vi "多参数数据插入.vi"(8 "error in (no error)":errorcluster caption="错误输入（无错误）", 9 "编号":string, 10 "columns enable":T1, 11 "data in":T2) -> (0 "error out":errorcluster)   [LabVIEW 2016, in "斯坦道多参数.lvlib"]
uses:
  <vilib>/Utility/sysdir.llb/System Directory Type.ctl
  <vilib>/addons/database/Auxilliary.llb/DB Tools Parameter Info.ctl
  <vilib>/addons/database/Auxilliary.llb/DB Tools DataTypes.ctl
  <vilib>/addons/database/Auxilliary.llb/DB Tools Parameter Dir.ctl
  <vilib>/addons/database/Auxilliary.llb/DB Tools Column Info.ctl
  <vilib>/addons/database/Auxilliary.llb/DB Tools Format Datetime String (Time Stamp).vi
  <vilib>/addons/database/Connection.llb/DB Tools Open Connec (String).vi
  <vilib>/addons/database/Connection.llb/Conn Execute.vi
  <vilib>/addons/database/Recordset.llb/Rec Destroy - Connection.vi
  <vilib>/addons/database/Command.llb/Cmd Set Parameter Value (C).vi
  <vilib>/addons/database/Command.llb/Cmd Execute.vi
  <vilib>/addons/database/Recordset.llb/Rec Destroy - Command.vi
  <vilib>/addons/database/Command.llb/Cmd Delete.vi
  <vilib>/addons/database/NI_Database_API.lvlib
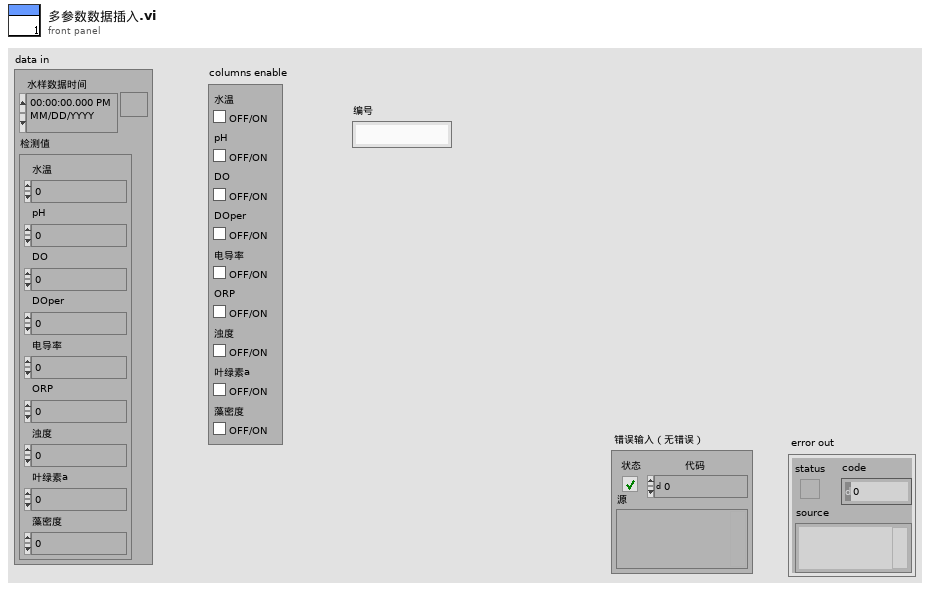
[diagram p1: front panel]
types:
  T1 = cluster{"水温":bool, "pH":bool, "DO":bool, "DOper":bool, "电导率":bool, "ORP":bool, "浊度":bool, "叶绿素a":bool, "藻密度":bool}
  T2 = cluster{"水样数据时间":timestamp, "检测值":cluster{"水温":dbl, "pH":dbl, "DO":dbl, "DOper":dbl, "电导率":dbl, "ORP":dbl, "浊度":dbl, "叶绿素a":dbl, "藻密度":dbl}}
  T3 = typedef "System Directory Type.ctl" = i32
  T4 = cluster{"水温":dbl, "pH":dbl, "DO":dbl, "DOper":dbl, "电导率":dbl, "ORP":dbl, "浊度":dbl, "叶绿素a":dbl, "藻密度":dbl}
  T5 = typedef "NI_Database_API.lvlib/DB Tools Column Info.ctl" = cluster{"column name":string, "data type":T6, "size":i32, "allow null?":bool}
  T6 = typedef "NI_Database_API.lvlib/DB Tools DataTypes.ctl" = enum16{"String", "Long (I32)", "Single (SGL)", "Double (DBL)", "Date/Time", "Binary"}
  T7 = typedef "NI_Database_API.lvlib/DB Tools Parameter Info.ctl" = cluster{"parameter name":string, "type":T6, "direction":T8, "value":variant}
  T8 = typedef "NI_Database_API.lvlib/DB Tools Parameter Dir.ctl" = enum32{"Input", "Output", "Input/Output", "Return Value"}
  T9 = typedef "NI_Database_API.lvlib/Conn ObjectReference.ctl" = refnum<k1>
  T10 = typedef "NI_Database_API.lvlib/Rec ObjectReference.ctl" = refnum<k1>
  T11 = typedef "NI_Database_API.lvlib/Cmd ObjectReference.ctl" = refnum<k1>
  T12 = typedef "NI_Database_API.lvlib/Cmd-Rec Object Reference.ctl" = refnum<k1>
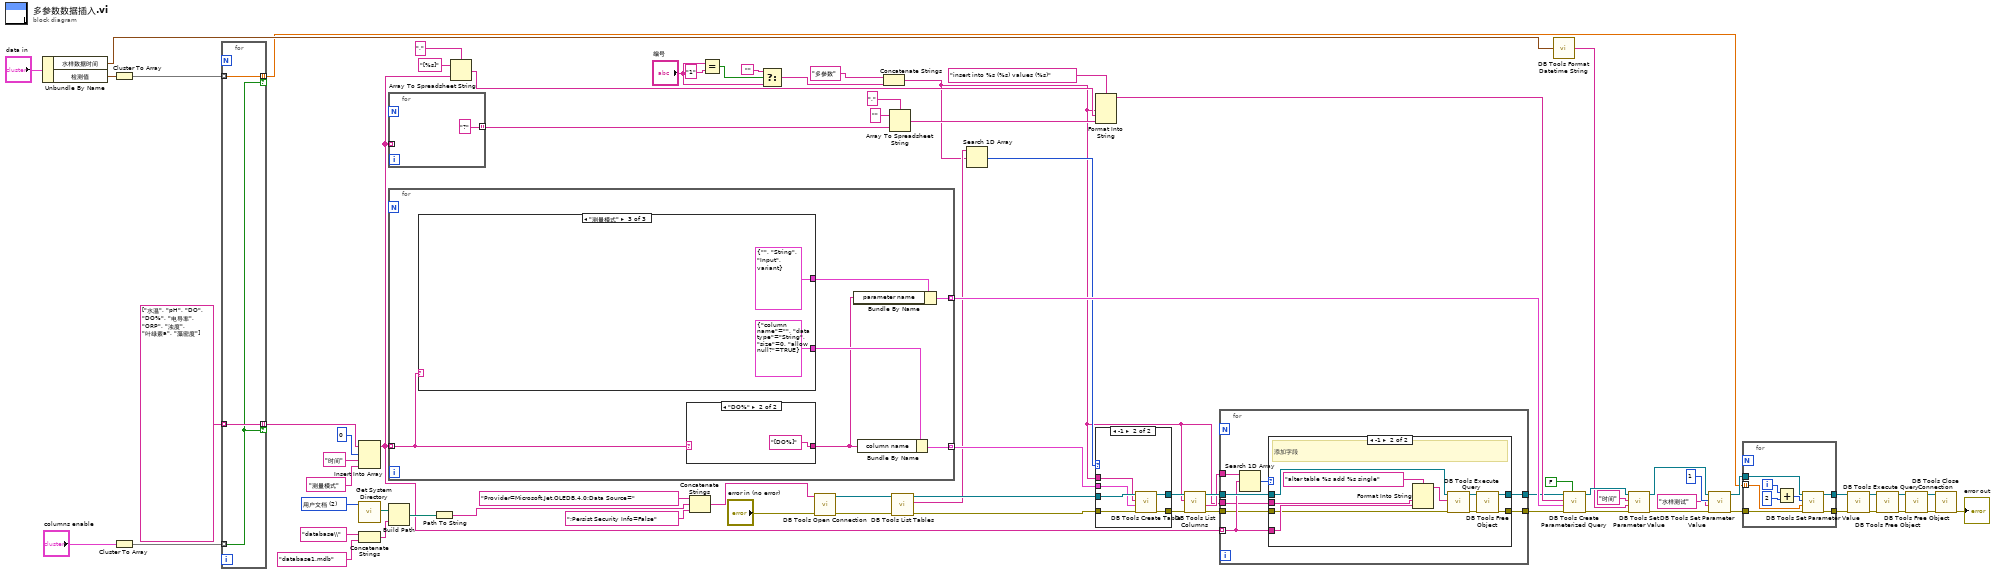
[diagram p0: block diagram]
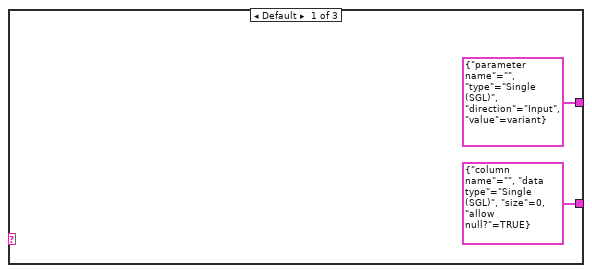
[diagram p5: hidden frame]
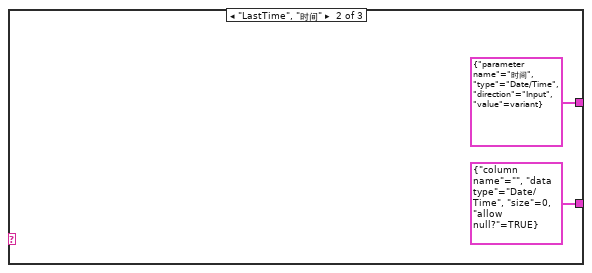
[diagram p6: hidden frame]
diagram:
  w75 = T3 2 items=["用户目录"=0, "用户桌面"=1, "用户文档"=2, "用户应用程序数据"=3, "用户设置"=4, "用户临时目录"=5, "公共文档"=6, "公共应用程序数据"=7, "公共设置"=8, "公共缓存"=13, "系统核心库"=9, "系统安装库"=10, "应用程序文件"=11, "启动盘根目录"=12] ("system directory type")
  n1 = Unbundle By Name("data in") -> ("水样数据时间"=w31:timestamp, "检测值"=w21:T4)
  n2 = Cluster To Array(cluster=w21) -> (array=w20:dbl[])
  n3 = Cluster To Array(cluster="columns enable") -> (array=w59:bool[])
  n4 = for {
    tunnel: string[] ["水温", "pH", "DO", "DO%", "电导率", "ORP", "浊度", "叶绿素a", "藻密度"] ("columns name") -> [w78] mode=indexing
    tunnel: w59 -> [w76] mode=indexing
    tunnel: [w78] -> w8 mode=indexing if=w76
    tunnel: w20 -> [w77] mode=indexing
    tunnel: [w77] -> w19 mode=indexing if=w76
  }
  n5 = Insert Into Array(array=w8, index=0 ("索引"), new element #1="时间" ("新元素/子数组"), new element #2="测量模式" ("新元素/子数组")) -> (w16:string[])
  n6 = call <vilib>:"Get System Directory.vi"("system directory type"=w75) -> ("system directory"=w73:path)  [unwired: 10 in]
  n7 = Concatenate Strings("database\\" ("condition"), "database1.mdb" ("字符串")) -> (w67:string)
  n8 = for {
    tunnel: w16 -> [_] mode=indexing
    tunnel: ["?"] -> w46 mode=indexing
  }
  n9 = for {
    tunnel: w16 -> [w81] mode=indexing
    tunnel: [w82] -> w44 mode=indexing
    tunnel: [w84] -> w43 mode=indexing
    n10 = case shown="\"测量模式\"" w81 {
      tunnel: [T7 {"parameter name"="", "type"=enum."Single (SGL)", "direction"=enum."Input", "value"=variant} ("parameter information") T7 {"parameter name"="时间", "type"=enum."Date/Time", "direction"=enum."Input", "value"=variant} ("parameter information") T7 {"parameter name"="", "type"=enum."String", "direction"=enum."Input", "value"=variant} ("parameter information")] -> w83
      tunnel: [T5 {"column name"="", "data type"=enum."Single (SGL)", "size"=0, "allow null?"=TRUE} ("column information") T5 {"column name"="", "data type"=enum."Date/Time", "size"=0, "allow null?"=TRUE} ("column information") T5 {"column name"="", "data type"=enum."String", "size"=0, "allow null?"=TRUE} ("column information")] -> w85
      frame Default {
      }
      frame "LastTime", "时间" {
      }
      frame "测量模式" {
      }
    }
    n11 = case shown="\"DO%\"" w81 {
      selector: w81 -> [w86 _]
      tunnel: [w86 "[DO%]"] -> w80
      frame "假", Default {
      }
      frame "DO%" {
      }
    }
    n12 = Bundle By Name(cluster=w83, "parameter name"=w80) -> (w82:T7)
    n13 = Bundle By Name(cluster=w85, "column name"=w80) -> (w84:T5)
  }
  n14 = Build Path(base path=w73, name or relative path=w67) -> (appended path=w72:path)
  n15 = Path To String(path=w72) -> (string=w71:string)
  n16 = Array To Spreadsheet String(delimiter (Tab)="," ("分隔符(Tab)"), array=w16, 3:"[%s]" ("格式字符串")) -> (spreadsheet string=w55:string)
  n17 = Concatenate Strings("Provider=Microsoft.Jet.OLEDB.4.0;Data Source=" ("condition"), w71, ";Persist Security Info=False" ("condition")) -> (w69:string)
  n18 = Equal?(x="编号", y="1") -> (x = y?=w4:bool)
  n19 = Select(t="", s=w4, f="编号") -> (s? t:f=w1:string)
  n20 = call-poly <vilib>:"DB Tools Open Connection.vi"("error in (no error)"="error in (no error)", "connection information"=w69) -> ("error out"=w63:errorcluster, "connection reference"=w65:T9)  [unwired: 6 in]
  n21 = Concatenate Strings("多参数" ("字符串"), w1) -> (w6:string)
  n22 = Array To Spreadsheet String(delimiter (Tab)="," ("分隔符(Tab)"), array=w46, 3:"" ("格式字符串")) -> (spreadsheet string=w50:string)
  n23 = call <vilib>:"DB Tools List Tables.vi"("error in (no error)"=w63, "connection reference"=w65) -> ("error out"=w42:errorcluster, "tables"=w40:string[], "connection reference out"=w45:T9)  [unwired: 3 in]
  n24 = Search 1D Array(1D array=w40, element=w6) -> (index of element=w39:i32)  [unwired: 1 in]
  n25 = Format Into String(format string="insert into %s (%s) values (%s)" ("格式字符串"), w6, w55, w50) -> (resulting string=w49:string)  [unwired: 2 in, 1 out]
  n26 = case shown="-1" w39 {
    tunnel: w45 -> [w95 w101]
    tunnel: [w95 w100] -> w15
    tunnel: [w94 w99] -> w13
    tunnel: w43 -> [_ w97]
    tunnel: w42 -> [w94 w98]
    tunnel: w6 -> [_ w96]
    frame 0, Default {
    }
    frame -1 {
      n27 = call <vilib>:"DB Tools Create Table.vi"("error in (no error)"=w98, "column information"=w97, "table"=w96, "connection reference"=w101) -> ("error out"=w99:errorcluster, "connection reference out"=w100:T9)  [unwired: 4 in]
    }
  }
  n28 = call <vilib>:"DB Tools List Columns.vi"("error in (no error)"=w13, "table"=w6, "connection reference"=w15) -> ("error out"=w11:errorcluster, "columns"=w12:string[], "connection reference out"=w14:T9)  [unwired: 1 in, 1 out]
  n29 = for {
    tunnel: w16 -> [w106] mode=indexing
    tunnel: w14 -> [w107]
    tunnel: w12 -> [w109]
    tunnel: w11 -> [w105]
    tunnel: [w104] -> w9
    tunnel: [w103] -> w10
    tunnel: w6 -> [w102]
    n30 = Search 1D Array(1D array=w109, element=w106) -> (index of element=w108:i32)  [unwired: 1 in]
    n31 = case shown="-1" w108 {
      tunnel: [w111 w117] -> w103
      tunnel: [w110 w116] -> w104
      tunnel: w107 -> [w111 w115]
      tunnel: w106 -> [_ w114]
      tunnel: w105 -> [w110 w113]
      tunnel: w102 -> [_ w112]
      frame 0, Default {
      }
      frame -1 {
        # "添加字段"
        n32 = Format Into String(format string="alter table %s add %s single", w112, w114) -> (resulting string=w118:string)  [unwired: 2 in, 1 out]
        n33 = call-poly <vilib>:"DB Tools Execute Query.vi"("error in (no error)"=w113, "SQL query"=w118, "connection reference"=w115) -> ("error out"=w120:errorcluster, "recordset reference"=w121:T10)  [unwired: 5 in]
        n34 = call-poly <vilib>:"DB Tools Free Object.vi"("error in (no error)"=w120, "recordset reference"=w121) -> ("error out"=w116:errorcluster, "connection reference"=w117:T9)  [unwired: 8 in]
      }
    }
  }
  n35 = call-poly <vilib>:"DB Tools Format Datetime String.vi"("time stamp"=w31) -> ("date/time string"=w30:string)
  n36 = call <vilib>:"DB Tools Create Parameterized Query.vi"("auto-detect parameters? (F)"=FALSE, "error in (no error)"=w9, "parameters"=w44, "SQL query"=w49, "connection reference"=w10) -> ("error out"=w48:errorcluster, "command reference"=w47:T11)  [unwired: 2 in, 1 out]
  n37 = call-poly <vilib>:"DB Tools Set Parameter Value.vi"("error in (no error)"=w48, "value"=w30, "parameter index"="时间", "command reference"=w47) -> ("error out"=w27:errorcluster, "command reference out"=w28:T11)  [unwired: 4 in]
  n38 = call-poly <vilib>:"DB Tools Set Parameter Value.vi"("error in (no error)"=w27, "value"="水样测试", "parameter index"=1, "command reference"=w28) -> ("error out"=w22:errorcluster, "command reference out"=w23:T11)  [unwired: 4 in]
  n39 = for {
    tunnel: w23 -> [w125]
    tunnel: w22 -> [w126]
    tunnel: w19 -> [w124] mode=indexing
    tunnel: [w123] -> w18
    tunnel: [w122] -> w17
    i -> [w129]
    n40 = Add(x=w129, y=2) -> (x+y=w127:i32)
    n41 = call-poly <vilib>:"DB Tools Set Parameter Value.vi"("error in (no error)"=w126, "value"=w124, "parameter index"=w127, "command reference"=w125) -> ("error out"=w122:errorcluster, "command reference out"=w123:T11)  [unwired: 4 in]
  }
  n42 = call-poly <vilib>:"DB Tools Execute Query.vi"("error in (no error)"=w17, "command reference"=w18) -> ("error out"=w36:errorcluster, "command-recordset reference"=w37:T12)  [unwired: 6 in]
  n43 = call-poly <vilib>:"DB Tools Free Object.vi"("error in (no error)"=w36, "command-recordset reference"=w37) -> ("error out"=w35:errorcluster, "command reference"=w34:T11)  [unwired: 8 in]
  n44 = call-poly <vilib>:"DB Tools Free Object.vi"("error in (no error)"=w35, "command reference"=w34) -> ("error out"=w32:errorcluster, "connection reference"=w33:T9)  [unwired: 8 in]
  n45 = call <vilib>:"DB Tools Close Connection.vi"("error in (no error)"=w32, "connection reference"=w33) -> ("error out"=→"error out":errorcluster)  [unwired: 5 in]
